vi "Feature Vector.vi"(8 "n":i32=3, 11 "state":dbl[](array[numeric])=[0.46211715726000974, 0.46211715726000974, 0.7071067811865475]) -> (3 "vector":dbl[](array[numeric])=[1.0, -0.6056998670788134, -0.26625534204141565, 0.11873171128012475, -0.8619805458075959, 0.9254712927602428, -0.9718055614729862, 0.40101101649098936, 0.4860209227015219, 0.11873171128012475, -0.8619805458075959, 0.9254712927602428, -0.9718055614729862, 0.40101101649098936, 0.4860209227015219, -0.3494999859705848, 0.9572059942679109, -0.8100591010196486, -0.9718055614729862, 0.40101101649098936, 0.4860209227015219, -0.3494999859705848, 0.9572059942679109, -0.8100591010196486, 0.8888120986196519, -0.17370960499694593, -0.678380329305727])   [LabVIEW 2017]
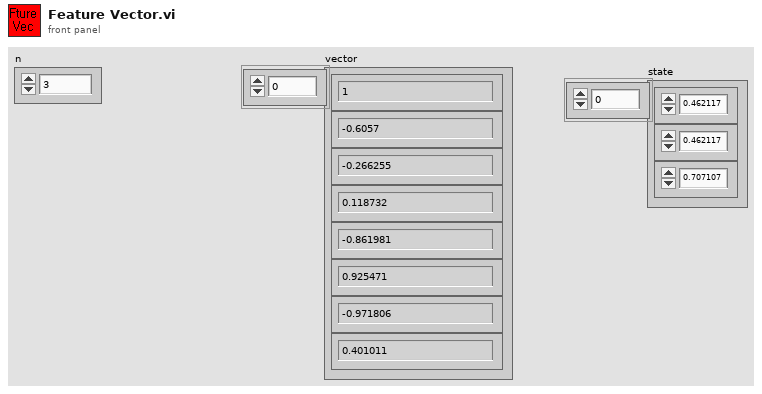
[diagram p1: front panel]
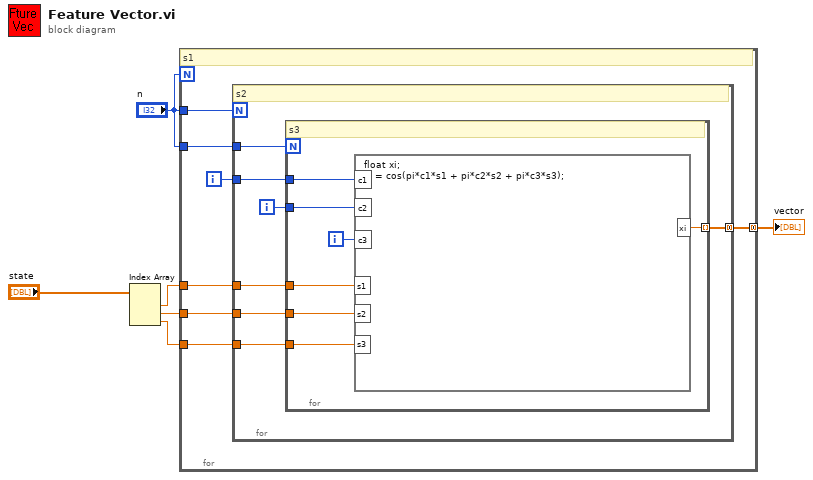
[diagram p0: block diagram]
diagram:
  n1 = Index Array(array="state") -> (element #1=w3:dbl, element #2=w2:dbl, element #3=w1:dbl)  [unwired: 3 in]
  n2 = for {
    N: "n" -> [_]
    tunnel: [w12] -> w6 mode=concatenating
    tunnel: "n" -> [w11]
    tunnel: "n" -> [w10]
    tunnel: w3 -> [w9]
    tunnel: w2 -> [w8]
    tunnel: w1 -> [w7]
    i -> [w13]
    # "s1"
    n3 = for {
      N: w11 -> [_]
      tunnel: w13 -> [w20]
      tunnel: [w18] -> w12 mode=concatenating
      tunnel: w10 -> [w17]
      tunnel: w9 -> [w16]
      tunnel: w8 -> [w15]
      tunnel: w7 -> [w14]
      i -> [w19]
      # "s2"
      n4 = for {
        N: w17 -> [_]
        tunnel: w20 -> [w27]
        tunnel: w19 -> [w26]
        tunnel: [w24] -> w18 mode=indexing
        tunnel: w16 -> [w23]
        tunnel: w15 -> [w22]
        tunnel: w14 -> [w21]
        i -> [w25]
        # "s3"
        n5 = formula code="float xi;\nxi = cos(pi*c1*s1 + pi*c2*s2 + pi*c3*s3);"("c1"=w27, "c2"=w26, "c3"=w25, "s1"=w23, "s2"=w22, "s3"=w21) -> ("xi"=w24:dbl)
      }
    }
  }
  "vector" <- w6
